vi "Producto Seleccionado.vi"(8 "error in (no error)":errorcluster, 10 "Producto Seleccionado":string, 11 "UI Actor in":refnum<class "UI Actor.lvclass">) -> (0 "error out":errorcluster, 3 "UI Actor out":refnum<class "UI Actor.lvclass">)   [LabVIEW 2019, in "UI Actor.lvlib" / "UI Actor.lvclass"]
uses:
  UI Actor.lvclass
  UI Actor.lvclass/UI Actor.ctl
  MENSAJES Messages/Actualiza Mensaje Msg/Actualiza Mensaje Msg.lvclass/Actualiza Mensaje Msg.ctl
  <vilib>/ActorFramework/Message Enqueuer/Message Enqueuer.lvclass/Message Enqueuer.ctl
  <vilib>/ActorFramework/Message Enqueuer/Enqueue.vi
  MENSAJES Messages/Actualiza Mensaje Msg/Actualiza Mensaje Msg.lvclass
  C:/Program Files (x86)/National Instruments/LabVIEW 2019/vi.lib/ActorFramework/Message/Message.lvclass
  <vilib>/ActorFramework/Message Priority Queue/Priority Enqueue.vi
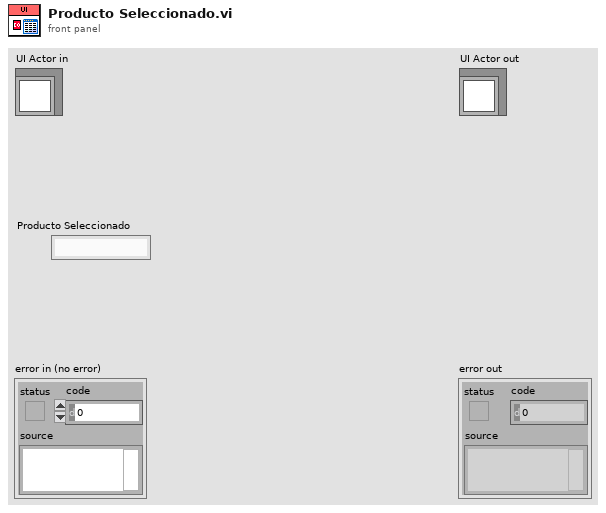
[diagram p1: front panel]
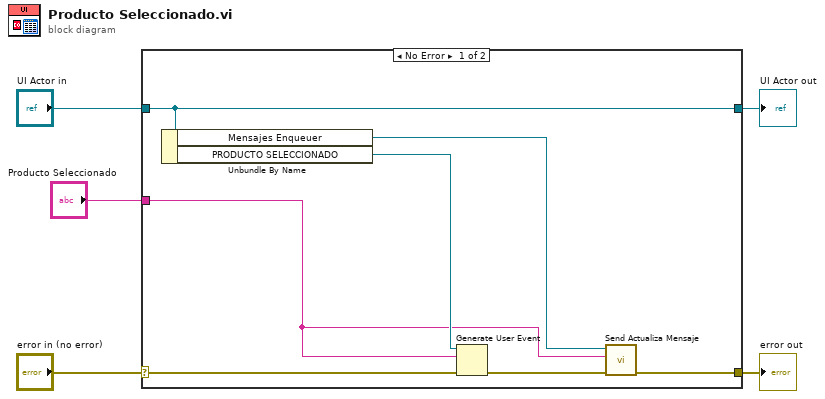
[diagram p0: block diagram]
diagram:
  n1 = case shown="No Error" "error in (no error)" {
    selector: "error in (no error)" -> [w11 w14]
    tunnel: [w8 w14] -> w4
    tunnel: [w12 w13] -> w2
    tunnel: "UI Actor in" -> [w12 w13]
    tunnel: "Producto Seleccionado" -> [w6 _]
    frame No Error {
      n2 = Unbundle By Name(w12) -> ("Mensajes Enqueuer"=w7:refnum<class "Message Enqueuer.lvclass">, "PRODUCTO SELECCIONADO"=w10:refnum<user-event>)
      n3 = Generate User Event(user event=w10, event data cluster=w6, error in=w11) -> (error out=w9:errorcluster)  [unwired: 1 in, 1 out]
      n4 = call "Send Actualiza Mensaje.vi"("error in (no error)"=w9, "Mensaje Status"=w6, "Message Enqueuer"=w7) -> ("error out"=w8:errorcluster)  [unwired: 7 in, 1 out]
    }
    frame Error {
    }
  }
  "error out" <- w4
  "UI Actor out" <- w2
